vi "Serial port is open.vi"(8 "error in (no error)":errorcluster, 11 "Serial Base in":refnum<class "Serial Base.lvclass">) -> (0 "error out":errorcluster, 2 "Is Port Connected?":bool, 3 "Serial Base out":refnum<class "Serial Base.lvclass">)   [LabVIEW 2022 SP3, in "Serial Base.lvclass"]
uses:
  Serial Base.lvclass
  Serial Base.lvclass/Serial Base.ctl
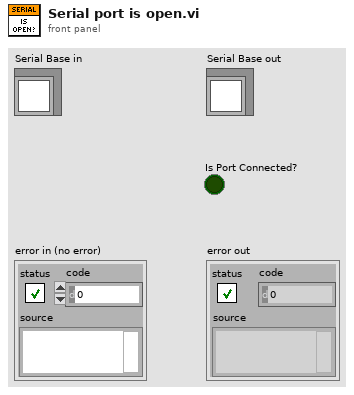
[diagram p1: front panel]
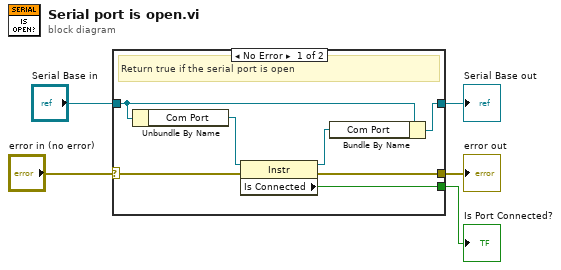
[diagram p0: block diagram]
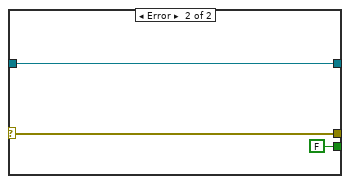
[diagram p2: hidden frame]
diagram:
  n1 = case shown="No Error" "error in (no error)" {
    selector: "error in (no error)" -> [w7 w15]
    tunnel: [w6 w15] -> w4
    tunnel: [w9 w14] -> w2
    tunnel: "Serial Base in" -> [w10 w14]
    tunnel: [w11 FALSE ("Is Connected")] -> w1
    frame No Error {
      # "Return true if the serial port is open"
      n2 = Unbundle By Name(w10) -> ("Com Port"=w12:refnum<visa-resource-name>)
      n3 = property class="Instr"(reference=w12, error in=w7) -> (reference out=w8:refnum<visa-resource-name>, error out=w6:errorcluster, "Is Connected"=w11:bool)
      n4 = Bundle By Name(cluster=w10, "Com Port"=w8) -> (w9:refnum<class "Serial Base.lvclass">)
    }
    frame Error {
    }
  }
  "error out" <- w4
  "Serial Base out" <- w2
  "Is Port Connected?" <- w1
